vi "SetVIAttribution.vi"(8 "error in (no error)":errorcluster caption="错误输入（无错误）", 11 "VI ref":refnum<vi>) -> (0 "error out":errorcluster caption="错误输出")   [LabVIEW 2018]
uses:
  Ctr/WindowAction.ctl
  Ctr/Reentry.ctl
  Ctr/Point.ctl
panel:
  in  "调用时清空显示控件":bool caption="Checkbox"
  in  "调用时挂起":bool caption="Checkbox"
  in  "运行时自动处理菜单":bool caption="Checkbox"
  in  "UseNowPosition":bool
  in  "坐标":T1
  in  "位置":u16(ring) items=["不改变", "居中", "最大化", "最小化", "自定义"]
  in  "调整窗口大小时缩放前面板上的对象":bool caption="Checkbox"
  in  "使用不同分辨率显示器时保持窗口比例":bool caption="Checkbox"
  in  "UseNowSize":bool
  in  "Height":i32 caption="高度"
  in  "Width":i32 caption="宽度"
  in  "高亮显示Enter布尔":bool caption="Checkbox"
  in  "窗口动作":T2
  in  "允许使用默认运行时快捷菜单":bool caption="Checkbox"
  in  "允许最小化窗口":bool caption="Checkbox"
  in  "允许调整窗口大小":bool caption="Checkbox"
  in  "允许关闭窗口":bool caption="Checkbox"
  in  "运行时透明显示窗口":bool caption="Checkbox"
  in  "如之前未打开则在运行后关闭":bool caption="Checkbox"
  in  "调用时显示前面板":bool caption="Checkbox"
  in  "显示连续运行按钮":bool caption="Checkbox"
  in  "显示运行按钮":bool caption="Checkbox"
  in  "显示终止按钮":bool caption="Checkbox"
  in  "运行时显示工具栏":bool caption="Checkbox"
  in  "显示水平滚动条":bool caption="Checkbox"
  in  "显示垂直滚动条":bool caption="Checkbox"
  in  "显示菜单栏":bool caption="Checkbox"
  in  "窗口包括标题栏":bool caption="Checkbox"
  in  "打开时运行":bool caption="Checkbox"
  in  "启用自动错误处理":bool caption="Checkbox"
  in  "重入":T3 caption="Checkbox"
  in  "在调用vi中内嵌子vi":bool caption="Checkbox"
  in  "允许调试":bool caption="Checkbox"
  in  "Transparency":u8 max=100
  # "执行"
  # "窗口外观"
  # "窗口尺寸"
  # "窗口位置"
  # "%"
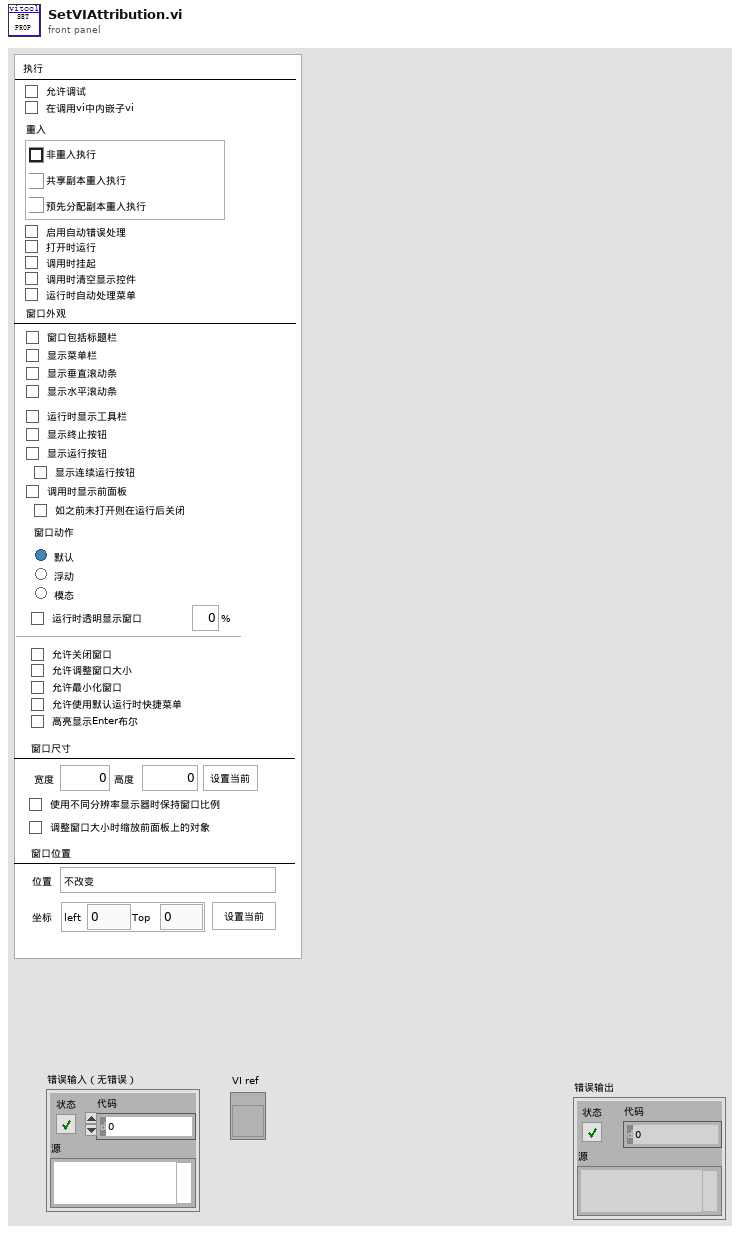
[diagram p1: front panel]
types:
  T1 = typedef "Point.ctl" = cluster{"left":dbl, "Top":dbl}
  T2 = typedef "WindowAction.ctl" = enum32{"Default", "Float", "Modal"}
  T3 = typedef "Reentry.ctl" = enum32{"非重入执行", "共享副本重入执行", "预先分配副本重入执行"}
  T4 = enum16{"Share clones between instances", "Preallocate clone for each instance"}
  T5 = enum32{"Invalid", "Default", "Floating", "Floating/Auto-Hide", "Modal"}
  T6 = enum16{"Always On", "Always Off", "Off While Running"}
  T7 = enum8{"Enabled", "Disabled", "Disabled and Grayed Out"}
  T8 = typedef "LVRectTypeDef.ctl" = cluster{"Left":i16, "Top":i16, "Right":i16, "Bottom":i16}
  T9 = typedef "LVPositionTypeDef.ctl" = cluster{"Left":i32, "Top":i32}
  T10 = typedef "LVBoundsTypeDef.ctl" = cluster{"Width":u32, "Height":u32}
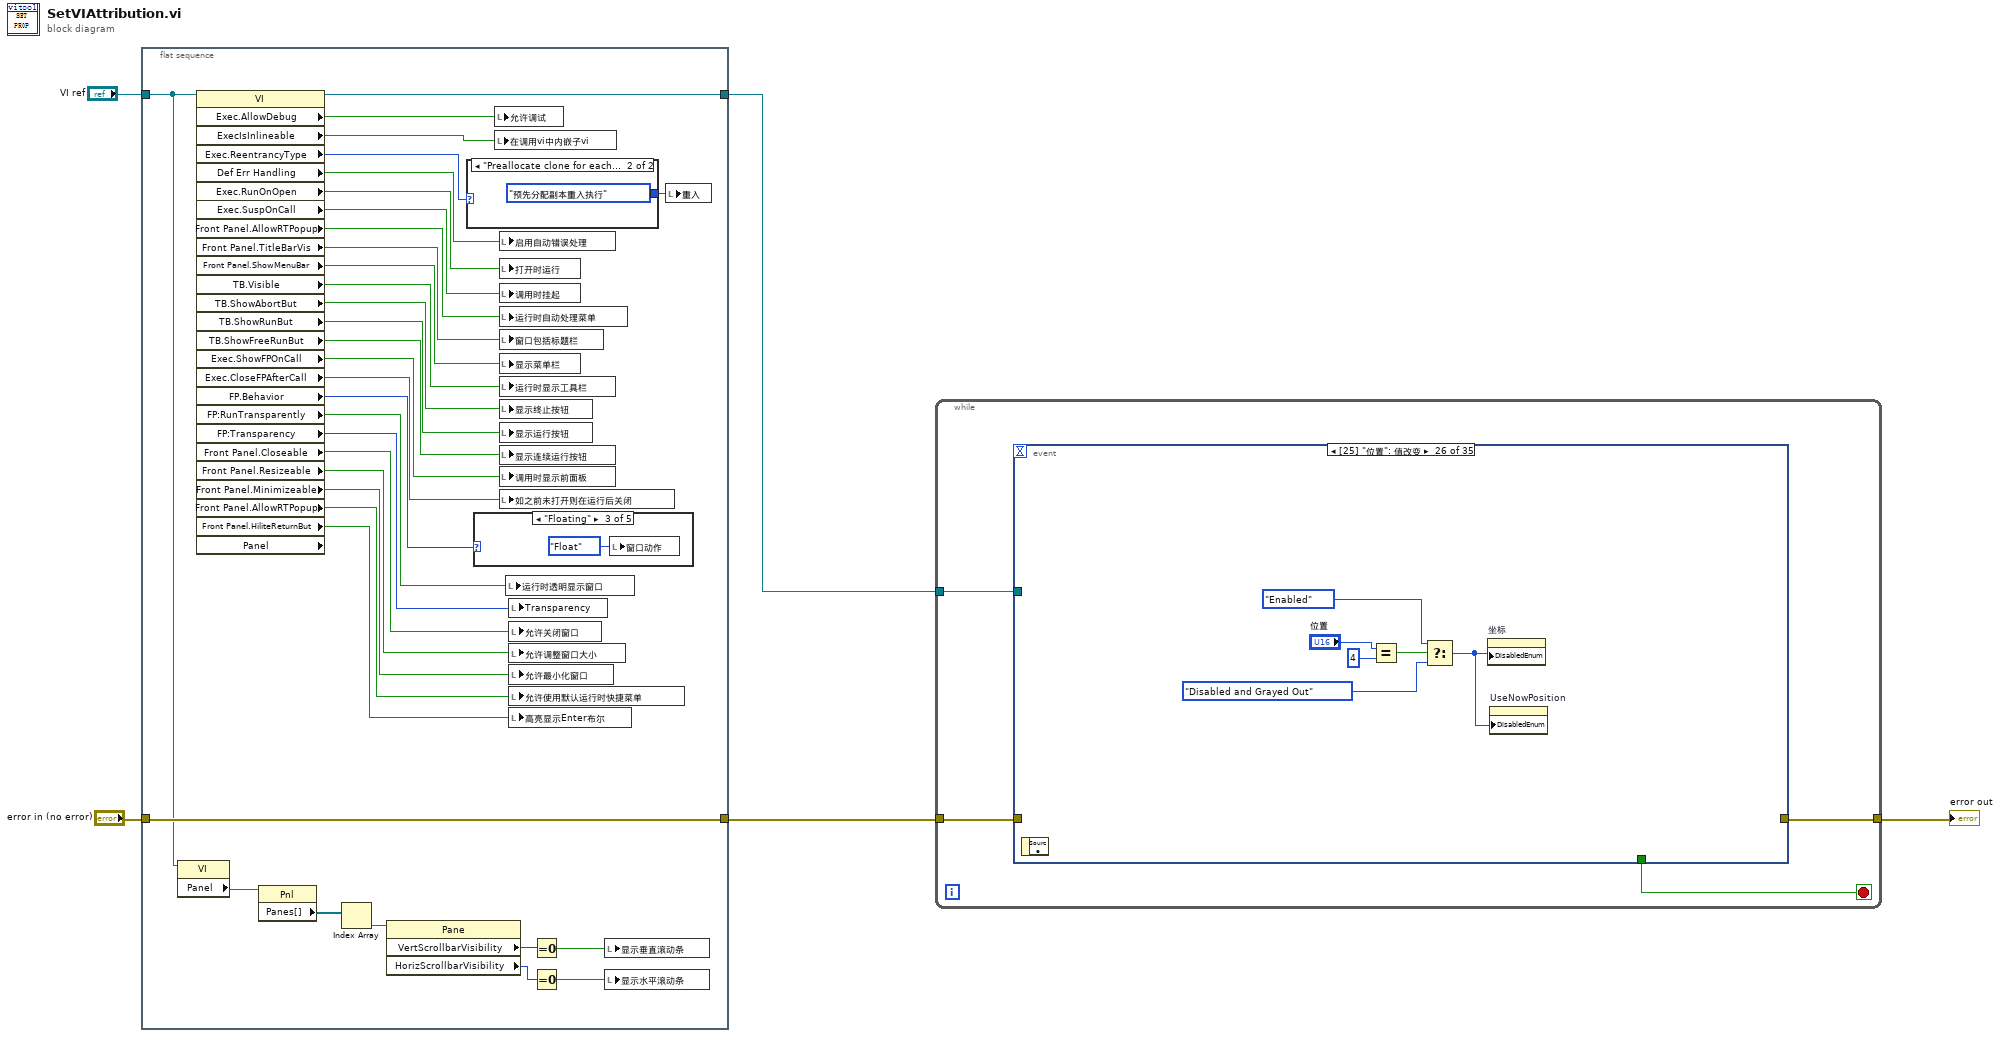
[diagram p0: block diagram]
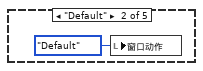
[diagram p3: hidden frame]
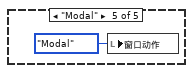
[diagram p5: hidden frame]
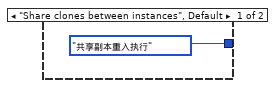
[diagram p6: hidden frame]
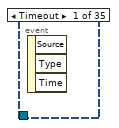
[diagram p7: hidden frame]
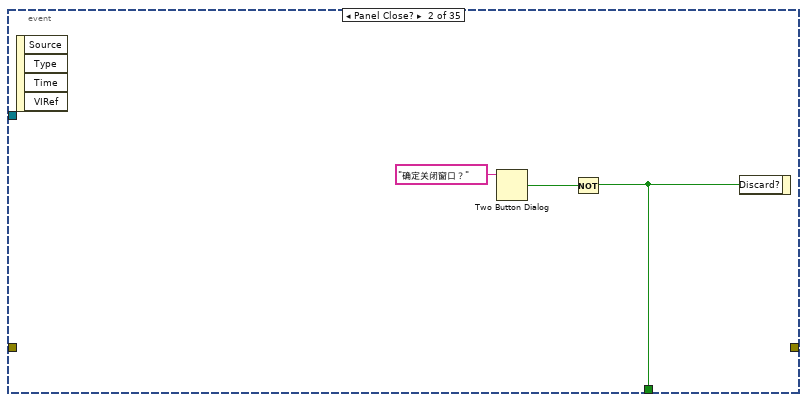
[diagram p8: hidden frame]
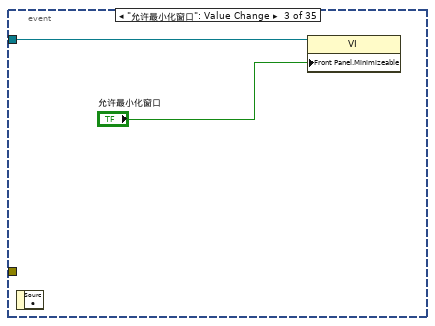
[diagram p9: hidden frame]
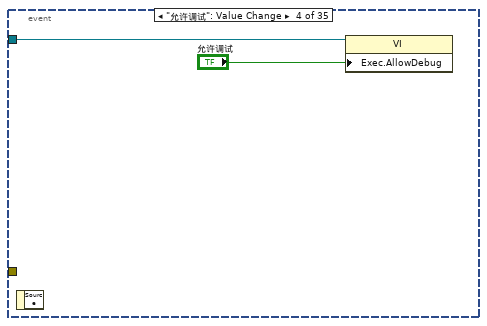
[diagram p10: hidden frame]
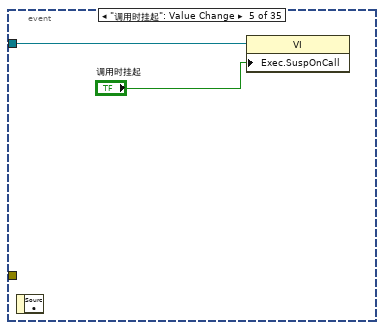
[diagram p11: hidden frame]
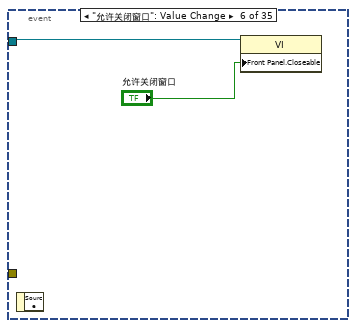
[diagram p12: hidden frame]
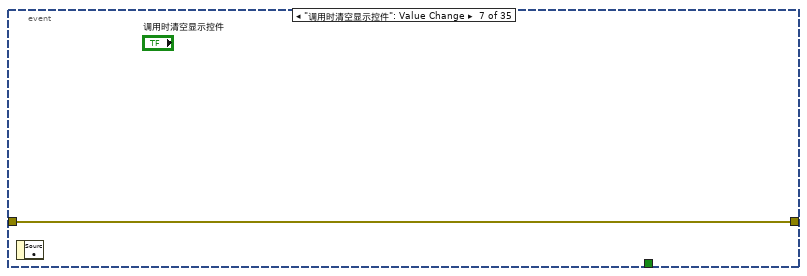
[diagram p13: hidden frame]
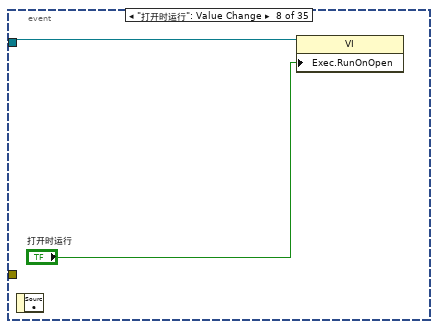
[diagram p14: hidden frame]
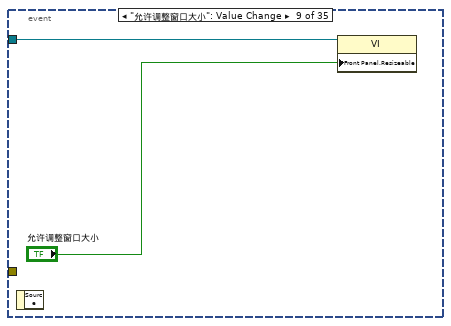
[diagram p15: hidden frame]
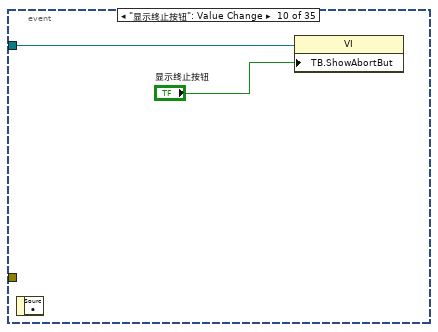
[diagram p16: hidden frame]
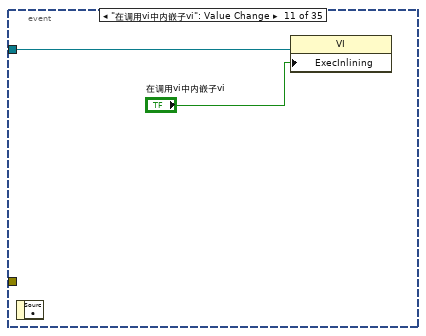
[diagram p17: hidden frame]
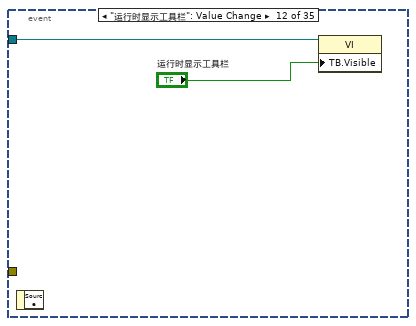
[diagram p18: hidden frame]
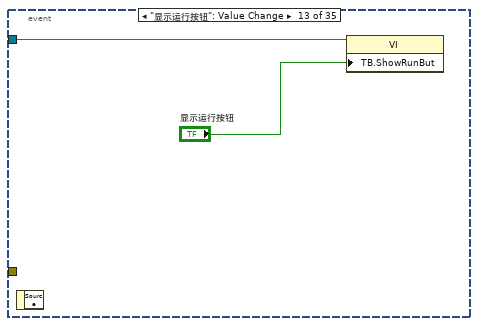
[diagram p19: hidden frame]
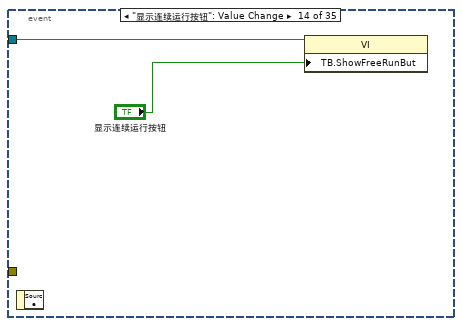
[diagram p20: hidden frame]
diagram:
  n1 = flat-sequence {
    tunnel: "VI ref" -> [w27]
    tunnel: [w39] -> w3
    tunnel: "error in (no error)" -> [w38]
    tunnel: [w38] -> w1
    frame #0 {
      n2 = property class="VI"(reference=w27) -> ("Panel"=w26:refnum<vi>)  [unwired: 1 in, 2 out]
      n3 = property class="VI" props=["Exec.AllowDebug", "ExecIsInlineable", "Exec.ReentrancyType", "Def Err Handling", "Exec.RunOnOpen", "Exec.SuspOnCall", "Front Panel.AllowRTPopup", "Front Panel.TitleBarVis", "Front Panel.ShowMenuBar", "TB.Visible", "TB.ShowAbortBut", "TB.ShowRunBut", "TB.ShowFreeRunBut", "Exec.ShowFPOnCall", "Exec.CloseFPAfterCall", "FP.Behavior", "FP:RunTransparently", "FP:Transparency", "Front Panel.Closeable", "Front Panel.Resizeable", "Front Panel.Minimizeable", "Front Panel.AllowRTPopup", "Front Panel.HiliteReturnBut", "Panel"](reference=w27) -> (reference out=w39:refnum<vi>, "Exec.AllowDebug"=w37:bool, "ExecIsInlineable"=w36:bool, "Exec.ReentrancyType"=w35:T4, "Def Err Handling"=w33:bool, "Exec.RunOnOpen"=w32:bool, "Exec.SuspOnCall"=w31:bool, "Front Panel.AllowRTPopup"=w30:bool, "Front Panel.TitleBarVis"=w29:bool, "Front Panel.ShowMenuBar"=w28:bool, "TB.Visible"=w19:bool, "TB.ShowAbortBut"=w18:bool, "TB.ShowRunBut"=w17:bool, "TB.ShowFreeRunBut"=w16:bool, "Exec.ShowFPOnCall"=w15:bool, "Exec.CloseFPAfterCall"=w14:bool, "FP.Behavior"=w13:T5, "FP:RunTransparently"=w12:bool, "FP:Transparency"=w11:u8, "Front Panel.Closeable"=w10:bool, "Front Panel.Resizeable"=w9:bool, "Front Panel.Minimizeable"=w8:bool, "Front Panel.AllowRTPopup"=w7:bool, "Front Panel.HiliteReturnBut"=w6:bool)  [unwired: 1 in, 2 out]
      n4 = property class="Pnl"(reference=w26) -> ("Panes[]"=w25:refnum<vi>[])  [unwired: 1 in, 2 out]
      n5 = Index Array(array=w25) -> (element=w24:refnum<vi>)  [unwired: 1 in]
      n6 = property class="Pane"(reference=w24) -> ("VertScrollbarVisibility"=w23:T6, "HorizScrollbarVisibility"=w21:T6)  [unwired: 1 in, 2 out]
      n7 = case shown="\"Preallocate clone for each instance\"" w35 {
        tunnel: [Reentry."共享副本重入执行" ("重入") Reentry."预先分配副本重入执行" ("重入")] -> w34
        frame "Share clones between instances", Default {
        }
        frame "Preallocate clone for each instance" {
        }
      }
      n8 = case shown="\"Floating\"" w13 {
        frame "Invalid", Default {
        }
        frame "Default" {
          n9 = local write "窗口动作"(WindowAction."Default" ("窗口动作")) -> ()
        }
        frame "Floating" {
          n10 = local write "窗口动作"(WindowAction."Float" ("窗口动作")) -> ()
        }
        frame "Floating/Auto-Hide" {
        }
        frame "Modal" {
          n11 = local write "窗口动作"(WindowAction."Modal" ("窗口动作")) -> ()
        }
      }
      n12 = local write "允许调试"(w37) -> ()
      n13 = local write "在调用vi中内嵌子vi"(w36) -> ()
      n14 = local write "启用自动错误处理"(w33) -> ()
      n15 = local write "打开时运行"(w32) -> ()
      n16 = local write "调用时挂起"(w31) -> ()
      n17 = local write "运行时自动处理菜单"(w30) -> ()
      n18 = local write "窗口包括标题栏"(w29) -> ()
      n19 = local write "显示菜单栏"(w28) -> ()
      n20 = local write "运行时显示工具栏"(w19) -> ()
      n21 = local write "显示终止按钮"(w18) -> ()
      n22 = local write "显示运行按钮"(w17) -> ()
      n23 = local write "显示连续运行按钮"(w16) -> ()
      n24 = local write "调用时显示前面板"(w15) -> ()
      n25 = local write "如之前未打开则在运行后关闭"(w14) -> ()
      n26 = local write "运行时透明显示窗口"(w12) -> ()
      n27 = local write "Transparency"(w11) -> ()
      n28 = local write "允许关闭窗口"(w10) -> ()
      n29 = local write "允许调整窗口大小"(w9) -> ()
      n30 = local write "允许最小化窗口"(w8) -> ()
      n31 = local write "允许使用默认运行时快捷菜单"(w7) -> ()
      n32 = local write "高亮显示Enter布尔"(w6) -> ()
      n33 = Equal To 0?(x=w23) -> (x = 0?=w22:bool)
      n34 = Equal To 0?(x=w21) -> (x = 0?=w20:bool)
      n35 = local write "显示垂直滚动条"(w22) -> ()
      n36 = local write "显示水平滚动条"(w20) -> ()
      n37 = local write "重入"(w34) -> ()
    }
  }
  n38 = while {
    tunnel: w3 -> [w47]
    tunnel: w1 -> [w46]
    tunnel: [w45] -> w5
    stop <- w48 stop-if-true
    n39 = event shown="[25] \"位置\": 值改变" {
      selector: _ -> [_ _ _ _ _ _ _ _ _ _ _ _ _ _ _ _ _ _ _ _ _ _ _ _ _ _ _ _ _ _ _ _ _ _ _]
      dyn-events: _ -> [_ _ _ _ _ _ _ _ _ _ _ _ _ _ _ _ _ _ _ _ _ _ _ _ _ _ _ _ _ _ _ _ _ _ _]
      timeout: _ -> [_ _ _ _ _ _ _ _ _ _ _ _ _ _ _ _ _ _ _ _ _ _ _ _ _ _ _ _ _ _ _ _ _ _ _]
      tunnel: [_ w50 _ _ _ _ _ _ _ _ _ _ _ _ _ _ _ _ _ _ _ _ _ _ _ _ _ _ _ _ _ _ _ _ _] -> w48
      tunnel: w47 -> [_ _ w53 w55 w57 w59 _ w62 w64 w66 w68 w70 w72 w74 w76 w78 w80 _ w82 w84 w86 w88 w89 w96 w110 _ w118 w121 w130 w135 w143 w146 w150 w156 _]
      tunnel: w46 -> [_ _ _ _ _ _ w60 _ _ _ _ _ _ _ _ _ _ _ _ _ _ _ w91 _ _ _ _ _ w129 w132 _ w145 w148 w152 w162]
      tunnel: [_ _ _ _ _ _ w60 _ _ _ _ _ _ _ _ _ _ _ _ _ _ _ w90 _ _ _ _ _ w125 w131 _ w144 w149 w157 w161] -> w45
      event Timeout {
        n40 = event-data() -> ()  [unwired: 1 in, 3 out]
      }
      event Panel Close? {
        n41 = event-data() -> ()  [unwired: 1 in, 4 out]
        n42 = Two Button Dialog(message="确定关闭窗口？" ("消息")) -> (T button?=w51:bool)  [unwired: 2 in]
        n43 = Not(x=w51) -> (.not. x?=w50:bool)
        n44 = event-data("Discard?"=w50) -> ()  [unwired: 1 in, 1 out]
      }
      event "允许最小化窗口": Value Change {
        n45 = event-data() -> ()  [unwired: 1 in, 1 out]
        n46 = property class="VI"(reference=w53, "Front Panel.Minimizeable"="允许最小化窗口") -> ()  [unwired: 1 in, 2 out]
      }
      event "允许调试": Value Change {
        n47 = event-data() -> ()  [unwired: 1 in, 1 out]
        n48 = property class="VI"(reference=w55, "Exec.AllowDebug"="允许调试") -> ()  [unwired: 1 in, 2 out]
      }
      event "调用时挂起": Value Change {
        n49 = event-data() -> ()  [unwired: 1 in, 1 out]
        n50 = property class="VI"(reference=w57, "Exec.SuspOnCall"="调用时挂起") -> ()  [unwired: 1 in, 2 out]
      }
      event "允许关闭窗口": Value Change {
        n51 = event-data() -> ()  [unwired: 1 in, 1 out]
        n52 = property class="VI"(reference=w59, "Front Panel.Closeable"="允许关闭窗口") -> ()  [unwired: 1 in, 2 out]
      }
      event "调用时清空显示控件": Value Change {
        n53 = event-data() -> ()  [unwired: 1 in, 1 out]
      }
      event "打开时运行": Value Change {
        n54 = event-data() -> ()  [unwired: 1 in, 1 out]
        n55 = property class="VI"(reference=w62, "Exec.RunOnOpen"="打开时运行") -> ()  [unwired: 1 in, 2 out]
      }
      event "允许调整窗口大小": Value Change {
        n56 = event-data() -> ()  [unwired: 1 in, 1 out]
        n57 = property class="VI"(reference=w64, "Front Panel.Resizeable"="允许调整窗口大小") -> ()  [unwired: 1 in, 2 out]
      }
      event "显示终止按钮": Value Change {
        n58 = event-data() -> ()  [unwired: 1 in, 1 out]
        n59 = property class="VI"(reference=w66, "TB.ShowAbortBut"="显示终止按钮") -> ()  [unwired: 1 in, 2 out]
      }
      event "在调用vi中内嵌子vi": Value Change {
        n60 = event-data() -> ()  [unwired: 1 in, 1 out]
        n61 = property class="VI"(reference=w68, "ExecInlining"="在调用vi中内嵌子vi") -> ()  [unwired: 1 in, 2 out]
      }
      event "运行时显示工具栏": Value Change {
        n62 = event-data() -> ()  [unwired: 1 in, 1 out]
        n63 = property class="VI"(reference=w70, "TB.Visible"="运行时显示工具栏") -> ()  [unwired: 1 in, 2 out]
      }
      event "显示运行按钮": Value Change {
        n64 = event-data() -> ()  [unwired: 1 in, 1 out]
        n65 = property class="VI"(reference=w72, "TB.ShowRunBut"="显示运行按钮") -> ()  [unwired: 1 in, 2 out]
      }
      event "显示连续运行按钮": Value Change {
        n66 = event-data() -> ()  [unwired: 1 in, 1 out]
        n67 = property class="VI"(reference=w74, "TB.ShowFreeRunBut"="显示连续运行按钮") -> ()  [unwired: 1 in, 2 out]
      }
      event "显示菜单栏": Value Change {
        n68 = event-data() -> ()  [unwired: 1 in, 1 out]
        n69 = property class="VI"(reference=w76, "Front Panel.ShowMenuBar"="显示菜单栏") -> ()  [unwired: 1 in, 2 out]
      }
      event "窗口包括标题栏": Value Change {
        n70 = event-data() -> ()  [unwired: 1 in, 1 out]
        n71 = property class="VI"(reference=w78, "Front Panel.TitleBarVis"="窗口包括标题栏") -> ()  [unwired: 1 in, 2 out]
      }
      event "调用时显示前面板": Value Change {
        n72 = event-data() -> ()  [unwired: 1 in, 1 out]
        n73 = property class="VI"(reference=w80, "Exec.ShowFPOnCall"="调用时显示前面板") -> ()  [unwired: 1 in, 2 out]
      }
      event "运行时自动处理菜单": Value Change {
        n74 = event-data() -> ()  [unwired: 1 in, 1 out]
      }
      event "启用自动错误处理": Value Change {
        n75 = event-data() -> ()  [unwired: 1 in, 1 out]
        n76 = property class="VI"(reference=w82, "Def Err Handling"="启用自动错误处理") -> ()  [unwired: 1 in, 2 out]
      }
      event "运行时透明显示窗口": Value Change {
        n77 = event-data() -> ()  [unwired: 1 in, 1 out]
        n78 = property class="VI"(reference=w84, "FP:RunTransparently"="运行时透明显示窗口") -> ()  [unwired: 1 in, 2 out]
      }
      event "Transparency": Value Change {
        n79 = event-data() -> ()  [unwired: 1 in, 1 out]
        n80 = property class="VI"(reference=w86, "FP:Transparency"="Transparency") -> ()  [unwired: 1 in, 2 out]
      }
      event "如之前未打开则在运行后关闭": Value Change {
        n81 = event-data() -> ()  [unwired: 1 in, 1 out]
        n82 = property class="VI"(reference=w88, "Exec.CloseFPAfterCall"="如之前未打开则在运行后关闭") -> ()  [unwired: 1 in, 2 out]
      }
      event "使用不同分辨率显示器时保持窗口比例": Value Change {
        n83 = event-data() -> ()  [unwired: 1 in, 1 out]
        n84 = property class="VI"(reference=w89, error in=w91, "Front Panel.KeepWinProps"="使用不同分辨率显示器时保持窗口比例") -> (error out=w90:errorcluster)  [unwired: 1 out]
      }
      event Value Change {
        n85 = event-data() -> ()  [unwired: 1 in, 1 out]
        n86 = Greater Than 0?(x="重入") -> (x > 0?=w95:bool)
        n87 = property class="VI"(reference=w96, "Exec.IsReentrant"=w95) -> (reference out=w93:refnum<vi>)  [unwired: 1 in, 1 out]
        n88 = case shown="\"预先分配副本重入执行\"" "重入" {
          tunnel: w93 -> [_ w98 w99]
          frame "非重入执行", Default {
          }
          frame "共享副本重入执行" {
            n89 = property class="VI"(reference=w98, "Exec.ReentrancyType"=0) -> ()  [unwired: 1 in, 2 out]
          }
          frame "预先分配副本重入执行" {
            n90 = property class="VI"(reference=w99, "Exec.ReentrancyType"=1) -> ()  [unwired: 1 in, 2 out]
          }
        }
      }
      event "Width", "Height": Value Change {
        n91 = event-data() -> ()  [unwired: 1 in, 1 out]
        n92 = property class="VI"(reference=w110) -> (reference out=w109:refnum<vi>, "Front Panel.WinBounds"=w107:T8)  [unwired: 1 in, 1 out]
        n93 = Unbundle By Name(w107) -> ("Left"=w108:i16, "Top"=w104:i16)
        n94 = Add(x=w108, y="Width") -> (x+y=w105:i32)
        n95 = Add(x=w104, y="Height") -> (x+y=w102:i32)
        n96 = Bundle By Name(cluster=w107, "Right"=w105, "Bottom"=w102) -> (w101:T8)
        n97 = property class="VI"(reference=w109, "Front Panel.WinBounds"=w101) -> ()  [unwired: 1 in, 2 out]
      }
      event "位置": Value Change {
        n98 = event-data() -> ()  [unwired: 1 in, 1 out]
        n99 = Equal?(x="位置", y=u16 4) -> (x = y?=w114:bool)
        n100 = Select(t=T7."Enabled" ("禁用"), s=w114, f=T7."Disabled and Grayed Out") -> (s? t:f=w111:T7)
        n101 = property on="坐标" class="Clust (严格)"("DisabledEnum"=w111) -> ()  [unwired: 2 in, 2 out]
        n102 = property on="UseNowPosition" class="Bool"("DisabledEnum"=w111) -> ()  [unwired: 2 in, 2 out]
      }
      event "高亮显示Enter布尔": Value Change {
        n103 = event-data() -> ()  [unwired: 1 in, 1 out]
        n104 = property class="VI"(reference=w118, "Front Panel.HiliteReturnBut"="高亮显示Enter布尔") -> ()  [unwired: 1 in, 2 out]
      }
      event Value Change {
        n105 = event-data() -> ()  [unwired: 1 in, 1 out]
        n106 = property class="VI"(reference=w121) -> ("Panel"=w120:refnum<vi>)  [unwired: 1 in, 2 out]
        n107 = local read "位置"() -> (w122:u16)
        n108 = case shown="4" w122 {
          tunnel: w120 -> [_ _ w124]
          tunnel: "坐标" -> [_ _ w123]
          frame 0, Default {
          }
          frame 1 {
          }
          frame 4 {
            n109 = property class="Pnl"(reference=w124, "Position"=w123) -> ()  [unwired: 1 in, 2 out]
          }
        }
      }
      event "UseNowPosition": Value Change {
        n110 = event-data() -> ()  [unwired: 1 in, 1 out]
        n111 = property class="VI"(reference=w130, error in=w129) -> (error out=w126:errorcluster, "Panel"=w128:refnum<vi>)  [unwired: 1 out]
        n112 = property class="Pnl"(reference=w128, error in=w126) -> (error out=w125:errorcluster, "Position"=w127:T9)  [unwired: 1 out]
        n113 = local write "坐标"(w127) -> ()
      }
      event Value Change {
        n114 = event-data() -> ()  [unwired: 1 in, 1 out]
        n115 = case shown="\"Float\"" "窗口动作" {
          tunnel: [T5."Default" ("前面板窗口:动作") T5."Floating" ("前面板窗口:动作") T5."Modal" ("前面板窗口:动作")] -> w133
          frame "Default", Default {
          }
          frame "Float" {
          }
          frame "Modal" {
          }
        }
        n116 = property class="VI"(reference=w135, error in=w132, "FP.Behavior"=w133) -> (error out=w131:errorcluster)  [unwired: 1 out]
      }
      event "UseNowSize": Value Change {
        n117 = event-data() -> ()  [unwired: 1 in, 1 out]
        n118 = property class="VI"(reference=w143) -> ("Panel"=w142:refnum<vi>)  [unwired: 1 in, 2 out]
        n119 = property class="Pnl"(reference=w142) -> ("Bounds"=w141:T10)  [unwired: 1 in, 2 out]
        n120 = Unbundle By Name(w141) -> ("Width"=w140:u32, "Height"=w139:u32)
        n121 = local write "Width"(w140) -> ()
        n122 = local write "Height"(w139) -> ()
      }
      event "调整窗口大小时缩放前面板上的对象": Value Change {
        n123 = event-data() -> ()  [unwired: 1 in, 1 out]
        n124 = property class="VI" props=["Panel"](reference=w146, error in=w145) -> (error out=w144:errorcluster)  [unwired: 2 out]
      }
      event "允许使用默认运行时快捷菜单": Value Change {
        n125 = event-data() -> ()  [unwired: 1 in, 1 out]
        n126 = property class="VI"(reference=w150, error in=w148, "Front Panel.AllowRTPopup"="允许使用默认运行时快捷菜单") -> (error out=w149:errorcluster)  [unwired: 1 out]
      }
      event "显示垂直滚动条": Value Change {
        n127 = event-data() -> ()  [unwired: 1 in, 1 out]
        n128 = property class="VI"(reference=w156) -> ("Panel"=w155:refnum<vi>)  [unwired: 1 in, 2 out]
        n129 = property class="Pnl"(reference=w155) -> ("Panes[]"=w154:refnum<vi>[])  [unwired: 1 in, 2 out]
        n130 = Select(t=T6."Always On" ("垂直滚动条可见"), s="显示垂直滚动条", f=T6."Always Off" ("垂直滚动条可见")) -> (s? t:f=w151:T6)
        n131 = Index Array(array=w154) -> (element=w153:refnum<vi>)  [unwired: 1 in]
        n132 = property on="属性节点" class="Pane"(reference=w153, error in=w152, "VertScrollbarVisibility"=w151) -> (error out=w157:errorcluster)  [unwired: 1 out]
      }
      event "显示水平滚动条": Value Change {
        n133 = event-data() -> ()  [unwired: 1 in, 1 out]
        n134 = Select(t=T6."Always On" ("水平滚动条可见"), s="显示水平滚动条", f=T6."Always Off") -> (s? t:f=w164:T6)
        n135 = property on="窗格" class="Pane"(error in=w162, "HorizScrollbarVisibility"=w164) -> (error out=w161:errorcluster)  [unwired: 1 in, 1 out]
      }
    }
  }
  "error out" <- w5
